vi "CODMn启动命令 (子VI).vi"(11 "启动测量模式":T1) -> ()   [LabVIEW 2016, in "斯坦道CODMn.lvlib"]
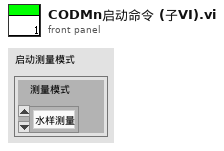
[diagram p1: front panel]
types:
  T1 = cluster{"测量模式":enum16{"水样测量", "标样核查", "零点核查", "跨度核查", "空白测试", "加标回收", "平行样", "校零", "校标"}}
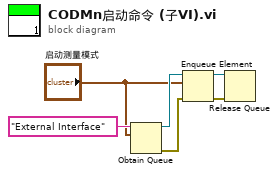
[diagram p0: block diagram]
diagram:
  n1 = Obtain Queue(name (unnamed)="External Interface" ("名称（未命名）"), element data type="启动测量模式") -> (queue out=w5:refnum<queue>, error out=w3:errorcluster)  [unwired: 3 in, 1 out]
  n2 = Enqueue Element(queue=w5, element="启动测量模式", error in (no error)=w3) -> (queue out=w2:refnum<queue>, error out=w1:errorcluster)  [unwired: 1 in, 1 out]
  n3 = Release Queue(queue=w2, error in (no error)=w1) -> ()  [unwired: 1 in, 3 out]
